vi "Feedback 適應性控制(雜訊消除).vi"() -> ()   [LabVIEW 2010]
uses:
  <vilib>/DAQmx/read.llb/DAQmx Read (Analog 1D DBL NChan 1Samp).vi
  <vilib>/DAQmx/write.llb/DAQmx Write (Analog DBL 1Chan 1Samp).vi
  <vilib>/DAQmx/create/channels.llb/DAQmx Create Channel (AI-Voltage-Basic).vi
  <vilib>/DAQmx/configure/timing.llb/DAQmx Timing (Sample Clock).vi
  <vilib>/DAQmx/create/channels.llb/DAQmx Create Channel (AO-Voltage-Basic).vi
  <vilib>/daqmx/miscellaneous.llb/DAQmx Fill In Error Info.vi
panel:
  in  "適應性雜訊消除":bool
  in  "u(收斂係數)":dbl=20.0
  in  "order":i32=1000
  in  "ch2-1估測DC時間(秒)":dbl=0.1
  in  "ch2-2 估測DC時間(秒)":dbl=0.1
  in  "ch2 Kii 增益":dbl
  in  "ch2 Kp 增益":dbl
  out "overload":bool
  in  "ch1 Kp 增益":dbl=-10.0
  in  "ch2 Ki 增益":dbl
  in  "ch1 Ki 增益":dbl=-500.0
  in  "ch1-2估測DC時間(秒)":dbl=2.0
  in  "ch2-3估測DC時間(秒)":dbl=0.1
  in  "Controller on":bool
  out "error out":errorcluster
  out "延遲百分比(%)  需小於0.5%":dbl=-0.0022542304036088368
  out "理想迴圈時間(ms)":dbl=0.16666666666666666
  out "迴圈平均運行時間(ms)":dbl=0.16666290961599398
  in  "output channels 1":tag="PXI-6733/ao0"
  in  "stop":bool
  in  "ch1-1估測DC時間(秒)":dbl=2.0
  in  "每通道取樣頻率(Hz)":dbl=6000.0 format="%0.2f"
  in  "input channels 2":tag="PXI-6229/ai1"
  in  "input channels 1":tag="PXI-6229/ai0"
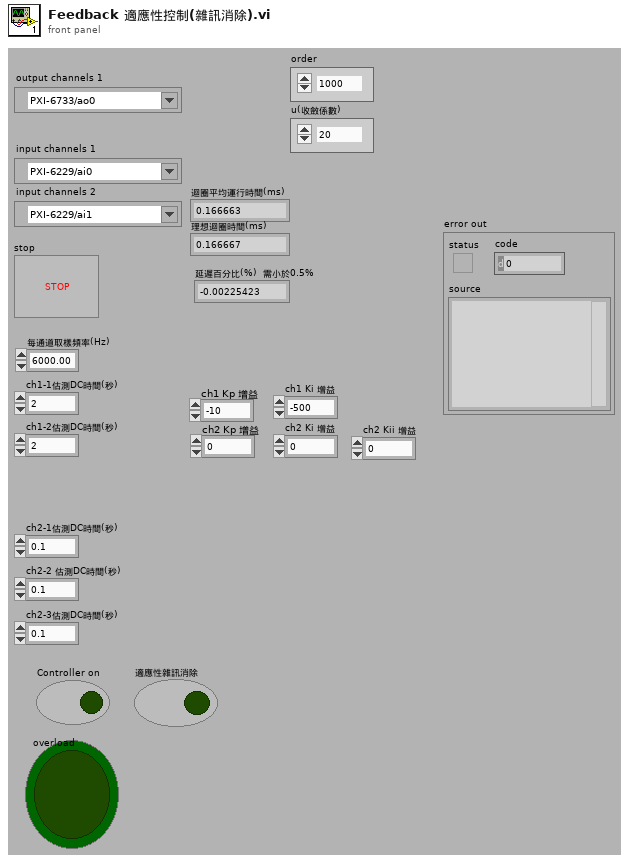
[diagram p1: front panel]
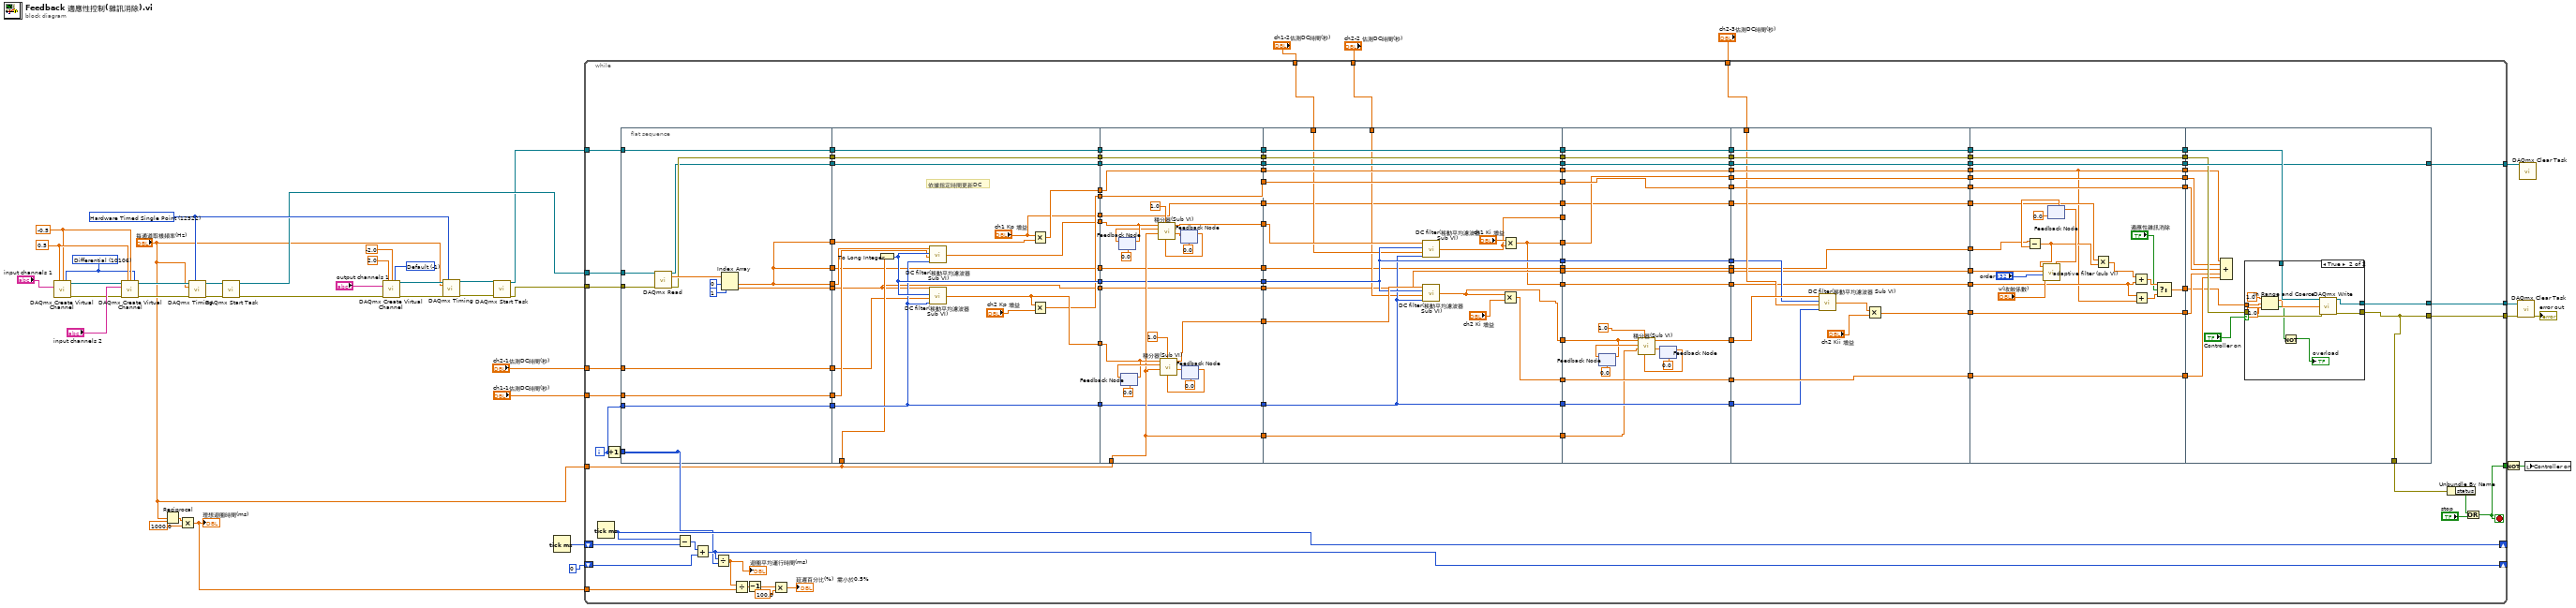
[diagram p0: block diagram]
diagram:
  w28 = -1 items=["Default"=-1, "RSE"=10083, "Differential"=10106, "Pseudodifferential"=12529] ("output terminal configuration")
  w25 = 12522 items=["Finite Samples"=10178, "Continuous Samples"=10123, "Hardware Timed Single Point"=12522] ("sample mode")
  w36 = 10106 items=["default"=-1, "RSE"=10083, "NRSE"=10078, "Differential"=10106, "Pseudodifferential"=12529] ("input terminal configuration")
  w37 = -0.5 ("minimum value")
  w38 = 0.5 ("maximum value")
  n1 = call-poly <vilib>:"DAQmx Create Virtual Channel.vi"("maximum value"=w38, "minimum value"=w37, "input terminal configuration"=w36, "physical channels"="input channels 1") -> ("task out"=w41:refnum<k21>, "error out"=w33:errorcluster)  [unwired: 10 in]
  n2 = call-poly <vilib>:"DAQmx Create Virtual Channel.vi"("task in"=w41, "maximum value"=w38, "minimum value"=w37, "input terminal configuration"=w36, "physical channels"="input channels 2", "error in"=w33) -> ("task out"=w35:refnum<k21>, "error out"=w32:errorcluster)  [unwired: 8 in]
  n3 = Reciprocal(x="每通道取樣頻率(Hz)") -> (1/x=w16:dbl)
  n4 = Multiply(x=w16, y=1000.0) -> (x*y=w14:dbl)
  "理想迴圈時間(ms)" <- w14
  n5 = call-poly <vilib>:"DAQmx Timing.vi"("task/channels in"=w35, "sample mode"=w25, "rate"="每通道取樣頻率(Hz)", "error in"=w32) -> ("task out"=w34:refnum<k21>, "error out"=w31:errorcluster)  [unwired: 10 in]
  n6 = call <vilib>:"DAQmx Start Task.vi"("task/channels in"=w34, "error in"=w31) -> ("task out"=w21:refnum<k21>, "error out"=w22:errorcluster)  [unwired: 12 in]
  n7 = call-poly <vilib>:"DAQmx Create Virtual Channel.vi"("maximum value"=2.0, "minimum value"=-2.0 ("maximum value"), "output terminal configuration"=w28, "physical channels"="output channels 1", "error in"=w22) -> ("task out"=w27:refnum<k21>, "error out"=w26:errorcluster)  [unwired: 9 in]
  n8 = call-poly <vilib>:"DAQmx Timing.vi"("task/channels in"=w27, "sample mode"=w25, "rate"="每通道取樣頻率(Hz)", "error in"=w26) -> ("task out"=w24:refnum<k21>, "error out"=w23:errorcluster)  [unwired: 10 in]
  n9 = call <vilib>:"DAQmx Start Task.vi"("task/channels in"=w24, "error in"=w23) -> ("task out"=w12:refnum<k21>, "error out"=w20:errorcluster)  [unwired: 12 in]
  n10 = Tick Count (ms)() -> (millisecond timer value=w18:u32)
  n11 = while {
    tunnel: w21 -> [w156]
    tunnel: w20 -> [w155]
    shift-right: [w152] -> _
    shift-left: w18 -> [w153]
    shift-right: [w149] -> _
    shift-left: 0 ("index") -> [w150]
    tunnel: w14 -> [w146]
    tunnel: "每通道取樣頻率(Hz)" -> [w103]
    tunnel: w12 -> [w133]
    tunnel: [w127] -> w9
    tunnel: [w101] -> w8
    tunnel: [w116] -> w7
    tunnel: "ch1-1估測DC時間(秒)" -> [w115]
    tunnel: [w102] -> w5
    tunnel: "ch1-2估測DC時間(秒)" -> [w85]
    tunnel: "ch2-3估測DC時間(秒)" -> [w84]
    tunnel: "ch2-2 估測DC時間(秒)" -> [w83]
    tunnel: "ch2-1估測DC時間(秒)" -> [w82]
    i -> [w113]
    stop <- w102 stop-if-true
    n12 = Tick Count (ms)() -> (millisecond timer value=w152:u32)
    n13 = Increment(x=w113) -> (x+1=w148:i32)
    n14 = flat-sequence {
      tunnel: w156 -> [w169]
      tunnel: w155 -> [w168]
      tunnel: [w157] -> w154
      tunnel: w148 -> [_]
      tunnel: w133 -> [w164]
      tunnel: [w164] -> w128
      tunnel: [w163] -> w126
      tunnel: [w162] -> w121
      tunnel: w115 -> [w161]
      tunnel: [w161] -> w114
      tunnel: w113 -> [w160]
      tunnel: [w160] -> w112
      tunnel: w82 -> [w159]
      tunnel: [w159] -> w81
      tunnel: [w157] -> w58
      tunnel: [w158] -> w57
      tunnel: [w157] -> w48
      tunnel: w154 -> [w184]
      tunnel: [w177] -> w141
      tunnel: [w174] -> w140
      tunnel: [w187] -> w129
      tunnel: w128 -> [w187]
      tunnel: w126 -> [w186]
      tunnel: [w186] -> w125
      tunnel: w121 -> [w185]
      tunnel: [w185] -> w117
      tunnel: w114 -> [w182]
      tunnel: w112 -> [w181]
      tunnel: [w183] -> w110
      tunnel: [w181] -> w108
      tunnel: w103 -> [w180]
      tunnel: [w179] -> w95
      tunnel: [w176] -> w91
      tunnel: w81 -> [w175]
      tunnel: [w173] -> w59
      tunnel: w58 -> [w173]
      tunnel: w57 -> [w172]
      tunnel: [w172] -> w56
      tunnel: w48 -> [w171]
      tunnel: ["ch1 Kp 增益"] -> w43
      tunnel: w141 -> [w203]
      tunnel: w140 -> [w214]
      tunnel: w103 -> [w200]
      tunnel: [w202] -> w139
      tunnel: [w201] -> w138
      tunnel: [w200] -> w135
      tunnel: [w199] -> w130
      tunnel: w129 -> [w199]
      tunnel: w125 -> [w198]
      tunnel: [w198] -> w123
      tunnel: [w197] -> w118
      tunnel: w117 -> [w197]
      tunnel: [w196] -> w111
      tunnel: w110 -> [w196]
      tunnel: [w195] -> w109
      tunnel: w108 -> [w195]
      tunnel: w95 -> [w192]
      tunnel: [w192] -> w92
      tunnel: w91 -> [w191]
      tunnel: [w191] -> w90
      tunnel: [w190] -> w60
      tunnel: w59 -> [w190]
      tunnel: w56 -> [w189]
      tunnel: [w189] -> w55
      tunnel: [w188] -> w44
      tunnel: w43 -> [w188]
      tunnel: w139 -> [w231]
      tunnel: w138 -> [w230]
      tunnel: [w223] -> w137
      tunnel: [w235] -> w136
      tunnel: w135 -> [w235]
      tunnel: [w234] -> w131
      tunnel: w130 -> [w234]
      tunnel: [w233] -> w124
      tunnel: w123 -> [w233]
      tunnel: [w232] -> w119
      tunnel: w118 -> [w232]
      tunnel: w111 -> [w229]
      tunnel: w109 -> [w228]
      tunnel: [w229] -> w106
      tunnel: [w228] -> w104
      tunnel: [w225] -> w93
      tunnel: w92 -> [w225]
      tunnel: w90 -> [w224]
      tunnel: [w224] -> w88
      tunnel: [w222] -> w87
      tunnel: [w216] -> w86
      tunnel: w85 -> [w221]
      tunnel: w83 -> [w220]
      tunnel: [w217] -> w64
      tunnel: [w219] -> w61
      tunnel: w60 -> [w219]
      tunnel: w55 -> [w218]
      tunnel: [w218] -> w54
      tunnel: [w216] -> w49
      tunnel: [w215] -> w45
      tunnel: w44 -> [w215]
      tunnel: w137 -> [w245]
      tunnel: w136 -> [w240]
      tunnel: [w252] -> w134
      tunnel: [w251] -> w132
      tunnel: w131 -> [w251]
      tunnel: w124 -> [w250]
      tunnel: [w250] -> w122
      tunnel: [w249] -> w120
      tunnel: w119 -> [w249]
      tunnel: [w248] -> w107
      tunnel: w106 -> [w248]
      tunnel: [w247] -> w105
      tunnel: w104 -> [w247]
      tunnel: [w241] -> w97
      tunnel: [w242] -> w96
      tunnel: [w244] -> w94
      tunnel: w93 -> [w244]
      tunnel: [w243] -> w89
      tunnel: w88 -> [w243]
      tunnel: w87 -> [w242]
      tunnel: w86 -> [w241]
      tunnel: w64 -> [_]
      tunnel: [w239] -> w62
      tunnel: w61 -> [w239]
      tunnel: w54 -> [w238]
      tunnel: [w238] -> w53
      tunnel: [w237] -> w50
      tunnel: w49 -> [w237]
      tunnel: [w236] -> w46
      tunnel: w45 -> [w236]
      tunnel: w134 -> [w272]
      tunnel: [w275] -> w80
      tunnel: w132 -> [w275]
      tunnel: [w274] -> w78
      tunnel: w122 -> [w274]
      tunnel: [w273] -> w76
      tunnel: w120 -> [w273]
      tunnel: w107 -> [w263]
      tunnel: w105 -> [w265]
      tunnel: w97 -> [w271]
      tunnel: [w271] -> w74
      tunnel: [w270] -> w72
      tunnel: w96 -> [w270]
      tunnel: [w269] -> w70
      tunnel: w94 -> [w269]
      tunnel: [w268] -> w68
      tunnel: w89 -> [w268]
      tunnel: [w266] -> w66
      tunnel: w84 -> [w264]
      tunnel: [w261] -> w63
      tunnel: w62 -> [w261]
      tunnel: w53 -> [w260]
      tunnel: [w260] -> w52
      tunnel: [w259] -> w51
      tunnel: w50 -> [w259]
      tunnel: [w258] -> w47
      tunnel: w46 -> [w258]
      tunnel: w80 -> [w298]
      tunnel: [w298] -> w79
      tunnel: w78 -> [w297]
      tunnel: [w297] -> w77
      tunnel: w76 -> [w296]
      tunnel: [w296] -> w75
      tunnel: w74 -> [w295]
      tunnel: [w295] -> w73
      tunnel: w72 -> [w294]
      tunnel: [w294] -> w71
      tunnel: w70 -> [w276]
      tunnel: [w276] -> w69
      tunnel: w68 -> [w293]
      tunnel: [w293] -> w67
      tunnel: w66 -> [w290]
      tunnel: [w290] -> w65
      tunnel: w63 -> [w277]
      tunnel: w52 -> [w286]
      tunnel: w51 -> [w283]
      tunnel: w47 -> [w282]
      tunnel: [w278] -> w42
      tunnel: w79 -> [w310]
      tunnel: [w309] -> w127
      tunnel: w77 -> [w306]
      tunnel: [w305] -> w101
      tunnel: [w308] -> w116
      tunnel: w75 -> [w308]
      tunnel: [w305] -> w100
      tunnel: w73 -> [w303]
      tunnel: w71 -> [w300]
      tunnel: w69 -> [w304]
      tunnel: w67 -> [w302]
      tunnel: w65 -> [w301]
      tunnel: w42 -> [w299]
      frame #0 {
        n15 = call-poly <vilib>:"DAQmx Read.vi"("task/channels in"=w169, "error in"=w168) -> ("task out"=w162:refnum<k21>, "data"=w165:dbl[], "error out"=w163:errorcluster)  [unwired: 11 in]
        n16 = Index Array(array=w165, index #1=0 ("index"), index #2=1 ("index")) -> (element #1=w157:dbl, element #2=w158:dbl)
      }
      frame #1 {
        # "依據指定時間更新DC"
        n17 = To Long Integer(number=w180) -> (32bit integer=w183:i32)
        n18 = call "DC filter(移動平均濾波器 Sub VI).vi"("當前迴圈計數(i)"=w181, "平均時間"=w175, "取樣頻率(Hz)"=w183, "input signal"=w172) -> ("DC filter output"=w177:dbl)
        n19 = call "DC filter(移動平均濾波器 Sub VI).vi"("當前迴圈計數(i)"=w181, "平均時間"=w182, "取樣頻率(Hz)"=w183, "input signal"=w184) -> ("DC filter output"=w174:dbl)
        n20 = Multiply(x="ch1 Kp 增益", y=w171) -> (x*y=w179:dbl)
        n21 = Multiply(x=w177, y="ch2 Kp 增益") -> (x*y=w176:dbl)
      }
      frame #2 {
        n22 = feedback #1(0.0) -> (w213:dbl)
        n23 = feedback-in #1(w214) -> ()
        n24 = feedback #2(0.0) -> (w204:dbl)
        n25 = feedback-in #2(w203) -> ()
        n26 = feedback #3(0.0 ("輸出累加ERR回朔")) -> (w211:dbl)
        n27 = call "積分器(Sub VI).vi"("輸入累加ERR回朔"=w211, "I增益"=1.0, "samples (Hz)"=w200, "前一個ERR"=w213, "當下ERR"=w214) -> ("輸出累加ERR回朔"=w212:dbl, "積分修正量"=w202:dbl)  [unwired: 5 in]
        n28 = feedback-in #3(w212) -> ()
        n29 = feedback #4(0.0 ("輸出累加ERR回朔")) -> (w206:dbl)
        n30 = call "積分器(Sub VI).vi"("輸入累加ERR回朔"=w206, "I增益"=1.0, "samples (Hz)"=w200, "前一個ERR"=w204, "當下ERR"=w203) -> ("輸出累加ERR回朔"=w205:dbl, "積分修正量"=w201:dbl)  [unwired: 5 in]
        n31 = feedback-in #4(w205) -> ()
      }
      frame #3 {
        n32 = call "DC filter(移動平均濾波器 Sub VI).vi"("當前迴圈計數(i)"=w228, "平均時間"=w221, "取樣頻率(Hz)"=w229, "input signal"=w231) -> ("DC filter output"=w217:dbl)
        n33 = call "DC filter(移動平均濾波器 Sub VI).vi"("當前迴圈計數(i)"=w228, "平均時間"=w220, "取樣頻率(Hz)"=w229, "input signal"=w230) -> ("DC filter output"=w223:dbl)
        n34 = Multiply(x=w223, y="ch2 Ki 增益") -> (x*y=w222:dbl)
        n35 = Multiply(x="ch1 Ki 增益", y=w217) -> (x*y=w216:dbl)
      }
      frame #4 {
        n36 = feedback #5(0.0) -> (w253:dbl)
        n37 = feedback-in #5(w245) -> ()
        n38 = feedback #6(0.0 ("輸出累加ERR回朔")) -> (w255:dbl)
        n39 = call "積分器(Sub VI).vi"("輸入累加ERR回朔"=w255, "I增益"=1.0, "samples (Hz)"=w240, "前一個ERR"=w253, "當下ERR"=w245) -> ("輸出累加ERR回朔"=w254:dbl, "積分修正量"=w252:dbl)  [unwired: 5 in]
        n40 = feedback-in #6(w254) -> ()
      }
      frame #5 {
        n41 = call "DC filter(移動平均濾波器 Sub VI).vi"("當前迴圈計數(i)"=w265, "平均時間"=w264, "取樣頻率(Hz)"=w263, "input signal"=w272) -> ("DC filter output"=w262:dbl)
        n42 = Multiply(x=w262, y="ch2 Kii 增益") -> (x*y=w266:dbl)
      }
      frame #6 {
        n43 = feedback #7(0.0 ("FIR輸出")) -> (w288:dbl)
        n44 = Subtract(x=w277, y=w288) -> (x-y=w284:dbl)
        n45 = call "adaptive filter (sub VI).vi"("ERR"=w284, "輸入訊號"=w286, "order"="order", "u(收斂係數)"="u(收斂係數)") -> ("FIR輸出"=w289:dbl)  [unwired: 3 in, 1 out]
        n46 = feedback-in #7(w289) -> ()
        n47 = Multiply(x=w282, y=w284) -> (x*y=w285:dbl)
        n48 = Add(x=w285, y=w283) -> (x+y=w281:dbl)
        n49 = Add(x=w283, y=w276) -> (x+y=w280:dbl)
        n50 = Select(t=w281, s="適應性雜訊消除", f=w280) -> (s? t:f=w278:dbl)
      }
      frame #7 {
        n51 = Compound Arithmetic op=ADD(w304, w303, w302, w301, w300) -> ()  [unwired: 1 out]
        n52 = case shown="True" "Controller on" {
          tunnel: w310 -> [_ w320]
          tunnel: [_ w319] -> w309
          tunnel: w306 -> [_ w318]
          tunnel: [_ w317] -> w305
          tunnel: w299 -> [_ w311]
          frame False {
          }
          frame True {
            n53 = In Range and Coerce(upper limit=1.0, x=w311, lower limit=-1.0) -> (coerced(x)=w316:dbl, In Range?=w313:bool)
            n54 = Not(x=w313) -> (.not. x?=→"overload":bool)
            n55 = call-poly <vilib>:"DAQmx Write.vi"("task/channels in"=w320, "data"=w316, "error in"=w318) -> ("task out"=w319:refnum<k21>, "error out"=w317:errorcluster)  [unwired: 10 in, 1 out]
          }
        }
      }
    }
    n56 = Subtract(x=w152, y=w153) -> (x-y=w151:u32)
    n57 = Add(x=w151, y=w150) -> (x+y=w149:u32)
    n58 = Divide(x=w149, y=w148) -> (x/y=w147:dbl)
    "迴圈平均運行時間(ms)" <- w147
    n59 = Divide(x=w147, y=w146) -> (x/y=w145:dbl)
    n60 = Decrement(x=w145) -> (x-1=w144:dbl)
    n61 = Multiply(x=w144, y=100.0) -> (x*y=→"延遲百分比(%)  需小於0.5%":dbl)
    n62 = Unbundle By Name(w100) -> ("status"=w99:bool)
    n63 = Or(x=w99, y="stop") -> (x .or. y?=w102:bool)
  }
  n64 = Not(x=w5) -> (.not. x?=w6:bool)
  n65 = call <vilib>:"DAQmx Clear Task.vi"("task in"=w9, "error in"=w8) -> ("error out"=→"error out":errorcluster)  [unwired: 13 in]
  n66 = call <vilib>:"DAQmx Clear Task.vi"("task in"=w7) -> ()  [unwired: 14 in, 1 out]
  n67 = local write "Controller on"(w6) -> ()
